vi "Initialize.vi"(8 "error in":errorcluster, 11 "Device Item Ref":T1 format="%.0x") -> (0 "error out":errorcluster, 3 "Device Item Ref out":T1 format="%.0x")   [LabVIEW 2020, in "Ballard ARINC 429 System Explorer.lvlib" / "Implementation.lvlib"]
uses:
  Implementation.lvlib
  <vilib>/NI VeriStand/Custom Device API/Custom Device Item Ref.ctl
  Scripting/Constants.vi
  <vilib>/NI VeriStand/Custom Device API/Set Item Property (Boolean).vi
  Scripting/Ballard ARINC 429 Scripting.lvlib
  <vilib>/NI VeriStand/Custom Device API/Custom Device API.lvlib
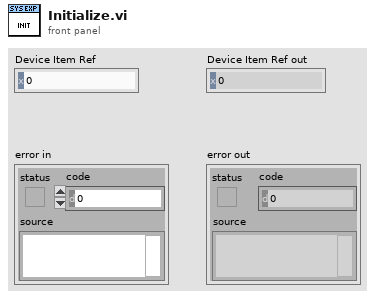
[diagram p1: front panel]
types:
  T1 = typedef "Custom Device API.lvlib/Custom Device Item Ref.ctl" = u64
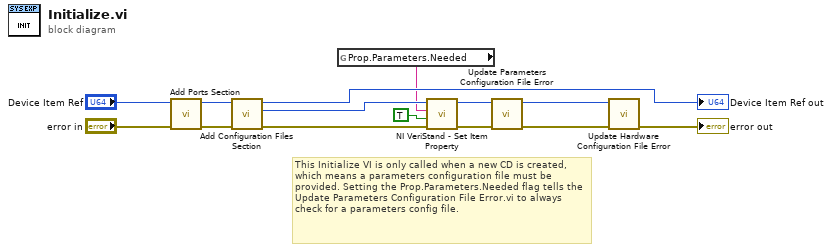
[diagram p0: block diagram]
diagram:
  # "This Initialize VI is only called when a new CD is created, which means a parameters configuration file must be provided. Setting the Prop.Parameters.Needed flag tells the Update Parameters Configuration File Error.vi to always check for a parameters config file."
  n1 = call "Add Ports Section.vi"("error in"="error in", "Custom device Ref"="Device Item Ref") -> ("error out"=w11:errorcluster, "Custom device Ref out"=w12:T1)  [unwired: 8 in]
  n2 = call "Add Configuration Files Section.vi"("error in"=w11, "Custom device Ref"=w12) -> ("error out"=w9:errorcluster, "Configuration files Ref"=w7:T1, "Custom device Ref out"=→"Device Item Ref out":T1)  [unwired: 7 in]
  n3 = global read "Constants.vi" "Prop.Parameters.Needed"() -> (w4:string)
  n4 = call-poly <vilib>:"NI VeriStand - Set Item Property.vi"("error in (no error)"=w9, "Value"=TRUE, "Property Name"=w4, "Item Ref in"=w7) -> ("error out"=w8:errorcluster, "Item Ref out"=w6:T1)  [unwired: 5 in, 1 out]
  n5 = call "Update Parameters Configuration File Error.vi"("error in"=w8, "Configuration files Ref"=w6) -> ("error out"=w3:errorcluster, "Configuration files Ref out"=w1:T1)  [unwired: 8 in]
  n6 = call "Update Hardware Configuration File Error.vi"("error in"=w3, "Configuration files Ref"=w1) -> ("error out"=→"error out":errorcluster)  [unwired: 8 in, 1 out]
